vi "Overwrite Decoration Content.vi"(8 "error in (no error)":errorcluster, 10 "Decos[]":refnum<vi>[](array[refnum]), 11 "Variant in":variant) -> (0 "error out":errorcluster, 3 "Variant out":variant)   [LabVIEW 2017, in "csmdoc.lvlib"]
uses:
  csmdoc.lvlib
  _Typedef/DocElement.ctl
  Communicable State Machine.lvlib
  _Shared/CSM Shared.lvlib
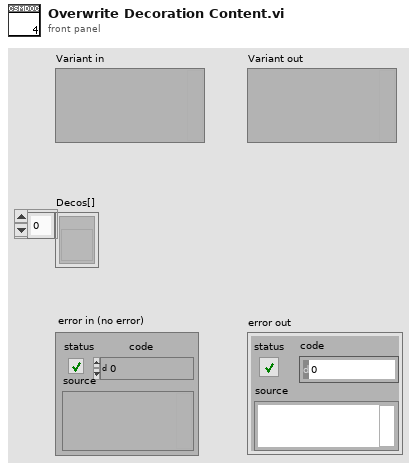
[diagram p1: front panel]
types:
  T1 = typedef "csmdoc.lvlib/DocElement.ctl" = cluster{"ID":string, "Content":string[], "SubIDs":string[], "Path":string[]}
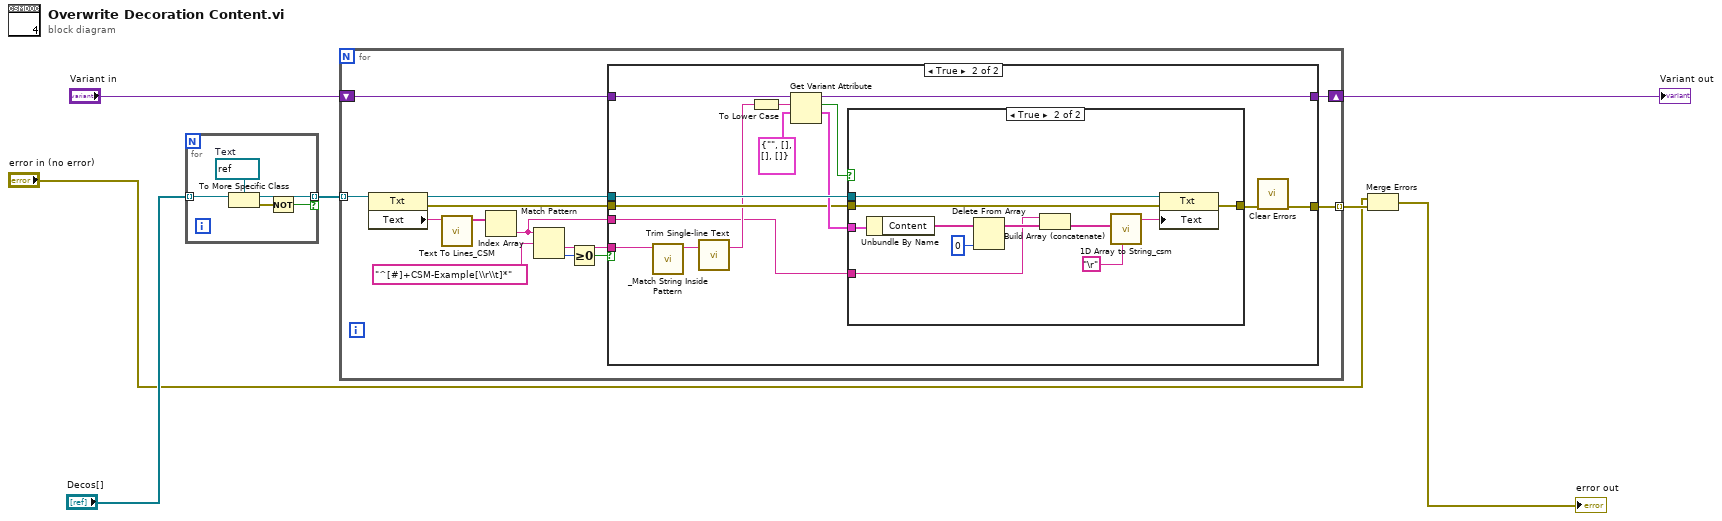
[diagram p0: block diagram]
diagram:
  n1 = for {
    tunnel: "Decos[]" -> [w12] mode=indexing
    tunnel: [w10] -> w3 mode=indexing if=w8
    w11 = refnum<vi> refnum  # Text
    n2 = To More Specific Class(target class=w11, reference=w12) -> (specific class reference=w10:refnum<vi>, error out=w9:errorcluster)  [unwired: 1 in]
    n3 = Not(x=w9) -> (.not. x?=w8:bool)
  }
  n4 = for {
    tunnel: w3 -> [w25] mode=indexing
    shift-right: [w21] -> w6
    shift-left: "Variant in" -> [w22]
    tunnel: [w18] -> w5 mode=indexing
    n5 = property class="Txt"(reference=w25) -> (reference out=w20:refnum<vi>, error out=w19:errorcluster, "Text"=w24:string)  [unwired: 1 in]
    n6 = call "Text To Lines_CSM.vi"("String"=w24) -> ("Lines"=w23:string[])  [unwired: 9 in, 1 out]
    n7 = Index Array(array=w23) -> (element=w15:string)  [unwired: 1 in]
    n8 = Match Pattern(string=w15, regular expression="^[#]+CSM-Example[\\r\\t]*") -> (after substring=w16:string, offset past match=w14:i32)  [unwired: 1 in, 2 out]
    n9 = Greater Or Equal To 0?(x=w14) -> (x >= 0?=w13:bool)
    n10 = case shown="True" w13 {
      tunnel: w22 -> [w26 w41]
      tunnel: [w26 w40] -> w21
      tunnel: w20 -> [_ w36]
      tunnel: w19 -> [w27 w33]
      tunnel: [w27 w31] -> w18
      tunnel: w16 -> [_ w30]
      tunnel: w15 -> [_ w28]
      frame False {
      }
      frame True {
        n11 = call "_Match String Inside Pattern.vi"("string"=w30) -> ("String inside"=w39:string)  [unwired: 10 in]
        n12 = call "Trim Single-line Text.vi"("single-line text"=w39) -> ("trimed text"=w29:string)  [unwired: 2 in]
        n13 = To Lower Case(string=w29) -> (all lower case string=w38:string)
        n14 = Get Variant Attribute(Variant=w41, name=w38, default value (empty Variant)=T1 {"ID"="", "Content"=[], "SubIDs"=[], "Path"=[]} ("Cluster")) -> (duplicate Variant=w40:variant, found=w35:bool, value=w34:T1)  [unwired: 1 in, 1 out]
        n15 = case shown="True" w35 {
          tunnel: w36 -> [_ w53]
          tunnel: w34 -> [_ w52]
          tunnel: w33 -> [w42 w49]
          tunnel: [w42 w48] -> w32
          tunnel: w28 -> [_ w43]
          frame False {
          }
          frame True {
            n16 = Unbundle By Name(w52) -> ("Content"=w47:string[])
            n17 = Delete From Array(array=w47, index=0) -> (array with subset deleted=w46:string[])  [unwired: 1 in, 1 out]
            n18 = Build Array (concatenate)(w43, w46) -> (w44:string[])
            n19 = call "1D Array to String_csm.vi"("delimiter (Tab)"="\r", "Array of Strings"=w44) -> ("delimited string"=w50:string)  [unwired: 9 in]
            n20 = property class="Txt"(reference=w53, error in=w49, "Text"=w50) -> (error out=w48:errorcluster)  [unwired: 1 out]
          }
        }
        n21 = call <vilib>:"Clear Errors.vi"("error in (no error)"=w32) -> ("error out"=w31:errorcluster)  [unwired: 5 in, 1 out]
      }
    }
  }
  "Variant out" <- w6
  n22 = Merge Errors("error in (no error)", w5) -> (→"error out":errorcluster)
